vi "TEST for feedback circuits-watch data.vi"() -> ()   [LabVIEW 2014]
uses:
  <vilib>/Analysis/baseanly.llb/Mean (DBL).vi
  <vilib>/Utility/file.llb/Read From Spreadsheet File (DBL).vi
  <vilib>/Analysis/NI_AALBase.lvlib
panel:
  in  "No feedback":path
  in  "Comp feedback":path
  out "XY Graph":cluster{dbl[], "all rows":dbl[]}[](graph)
  in  "Avg points":i32=50
  in  "Filter type":T1(ring)
  in  "Sampling rate (Hz)":dbl=200000.0
  in  "circuit feedback":path
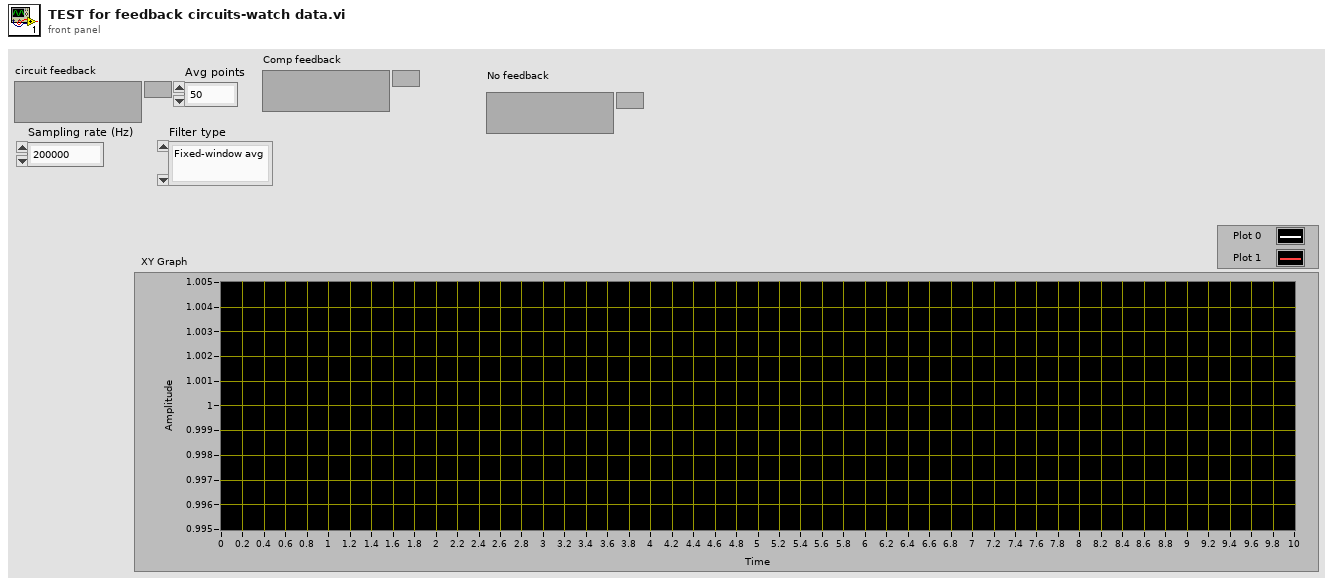
[diagram p1: front panel]
types:
  T1 = enum16{"Fixed-window avg", "Moving-window avg", "S-G filter", "Fixed-window Median", "Moving-window Median "}
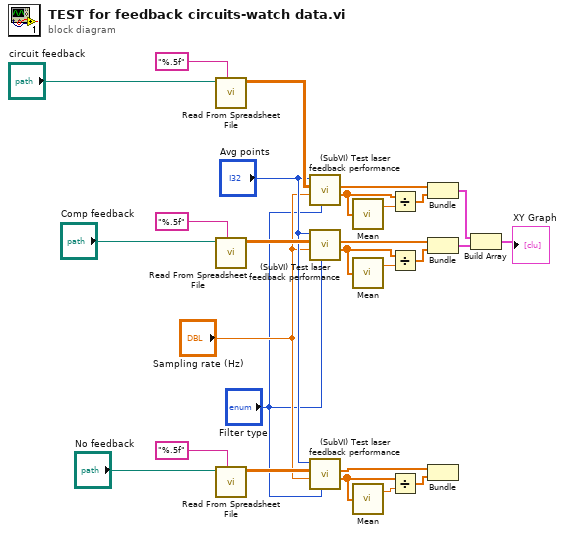
[diagram p0: block diagram]
diagram:
  n1 = call-poly <vilib>:"Read From Spreadsheet File.vi"("format (%.3f)"="%.5f", "file path (dialog if empty)"="circuit feedback") -> ("all rows"=w26:dbl[][])  [unwired: 5 in, 4 out]
  n2 = call-poly <vilib>:"Read From Spreadsheet File.vi"("format (%.3f)"="%.5f", "file path (dialog if empty)"="Comp feedback") -> ("all rows"=w22:dbl[][])  [unwired: 5 in, 4 out]
  n3 = call-poly <vilib>:"Read From Spreadsheet File.vi"("format (%.3f)"="%.5f", "file path (dialog if empty)"="No feedback") -> ("all rows"=w17:dbl[][])  [unwired: 5 in, 4 out]
  n4 = call "(SubVI) Test laser feedback performance .vi"("Filter type"="Filter type", "Sampling rate (Hz)"="Sampling rate (Hz)", "all rows"=w26, "Avg points"="Avg points") -> ("Filtered QPD data"=w8:dbl[], "Time"=w21:dbl[])  [unwired: 4 in, 2 out]
  n5 = call "(SubVI) Test laser feedback performance .vi"("Filter type"="Filter type", "Sampling rate (Hz)"="Sampling rate (Hz)", "all rows"=w22, "Avg points"="Avg points") -> ("Filtered QPD data"=w5:dbl[], "Time"=w13:dbl[])  [unwired: 4 in, 2 out]
  n6 = call "(SubVI) Test laser feedback performance .vi"("Filter type"="Filter type", "Sampling rate (Hz)"="Sampling rate (Hz)", "all rows"=w17, "Avg points"="Avg points") -> ("Filtered QPD data"=w2:dbl[], "Time"=w14:dbl[])  [unwired: 4 in, 2 out]
  n7 = call-poly <vilib>:"Mean.vi"("X"=w8) -> ("mean"=w9:dbl)  [unwired: 1 out]
  n8 = call-poly <vilib>:"Mean.vi"("X"=w5) -> ("mean"=w6:dbl)  [unwired: 1 out]
  n9 = call-poly <vilib>:"Mean.vi"("X"=w2) -> ("mean"=w3:dbl)  [unwired: 1 out]
  n10 = Divide(x=w8, y=w9) -> (x/y=w7:dbl[])
  n11 = Divide(x=w5, y=w6) -> (x/y=w4:dbl[])
  n12 = Divide(x=w2, y=w3) -> (x/y=w1:dbl[])
  n13 = Bundle("Time"=w21, w7) -> (w11:cluster{"Time ":dbl[], dbl[]})  [unwired: 1 in]
  n14 = Bundle("Time"=w13, w4) -> (w12:cluster{"Time ":dbl[], dbl[]})  [unwired: 1 in]
  n15 = Bundle("Time"=w14, w1) -> ()  [unwired: 1 in, 1 out]
  n16 = Build Array(w11, w12) -> (→"XY Graph":cluster{"Time ":dbl[], dbl[]}[])
